vi "LV Image to PNG Data Wrapper.vi"(8 "error in (no error)":errorcluster, 11 "image data":T1) -> (0 "error out":errorcluster, 3 "png data":string)   [LabVIEW 2011]
uses:
  <vilib>/picture/picture.llb/imagedata.ctl
  <vilib>/wsapi/NI_WebServices.lvlib
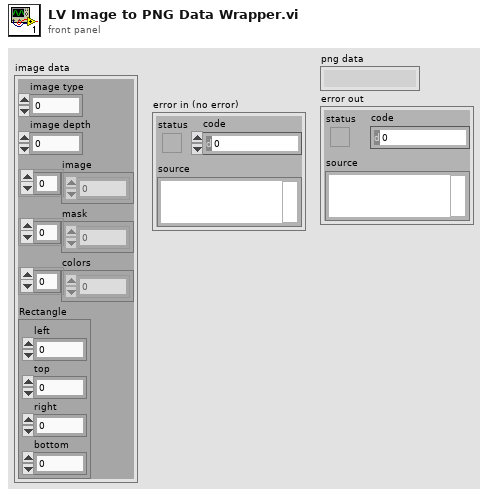
[diagram p1: front panel]
types:
  T1 = typedef "imagedata.ctl" = cluster{"image type":i32, "image depth":i32, "image":u8[], "mask":u8[], "colors":u32[], "Rectangle":cluster{"left":i16, "top":i16, "right":i16, "bottom":i16}}
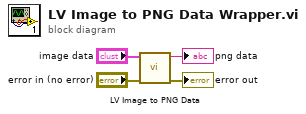
[diagram p0: block diagram]
diagram:
  n1 = call <vilib>:"LV Image to PNG Data.vi"("error in (no error)"="error in (no error)", "image data"="image data") -> ("error out"=→"error out":errorcluster, "png data"=→"png data":string)  [unwired: 8 in]
